vi "CalVision.vi"(10 "SerialPortIn":T1) -> (3 "SerialPortOut":T1)   [LabVIEW 2017, in "VisionHW.lvlib"]
uses:
  VisionHW.lvlib
  <vilib>/Rock Robotics/WPI/SerialPort/WPI_SerialPortRef.ctl
panel:
  out "Command":string
  in  "V Range":cluster{dbl, dbl}(slide) scale=0.0..255.0
  in  "S Range":cluster{dbl, dbl}(slide) scale=0.0..255.0
  in  "H Range":cluster{dbl, dbl}(slide) scale=0.0..255.0
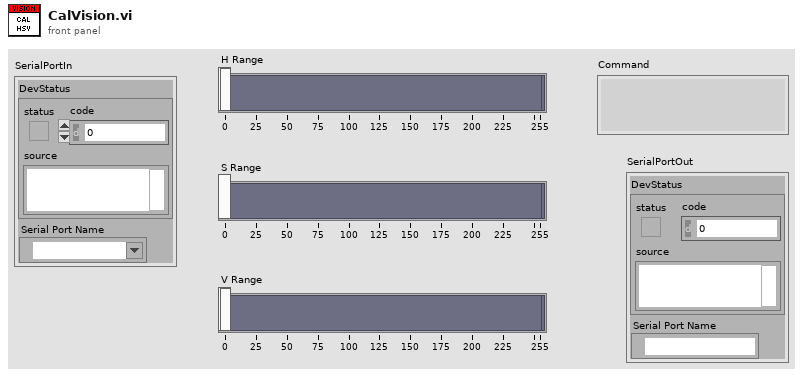
[diagram p1: front panel]
types:
  T1 = typedef "WPI_SerialPortRef.ctl" = cluster{"DevStatus":errorcluster, "Serial Port Name":refnum<visa-resource-name>}
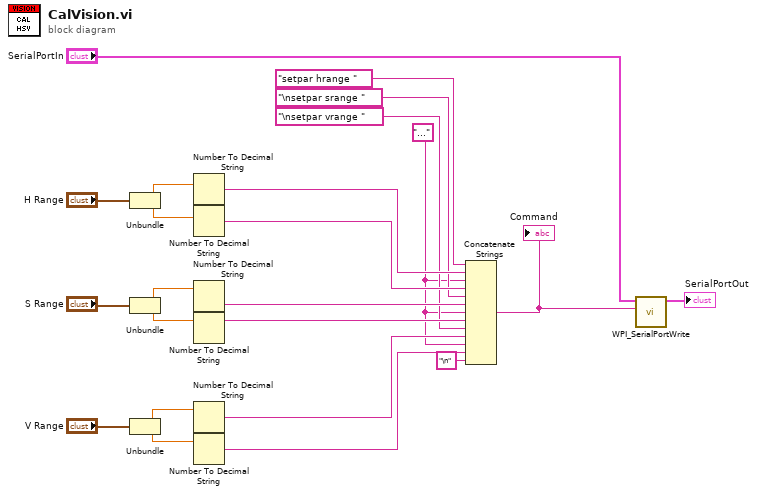
[diagram p0: block diagram]
diagram:
  w6 = "..." ("string")
  n1 = Unbundle("H Range") -> (w22:dbl, w19:dbl)
  n2 = Unbundle("S Range") -> (w15:dbl, w14:dbl)
  n3 = Unbundle("V Range") -> (w13:dbl, w12:dbl)
  n4 = Number To Decimal String(number=w22) -> (decimal integer string=w20:string)  [unwired: 1 in]
  n5 = Number To Decimal String(number=w19) -> (decimal integer string=w18:string)  [unwired: 1 in]
  n6 = Number To Decimal String(number=w15) -> (decimal integer string=w10:string)  [unwired: 1 in]
  n7 = Number To Decimal String(number=w14) -> (decimal integer string=w9:string)  [unwired: 1 in]
  n8 = Number To Decimal String(number=w13) -> (decimal integer string=w7:string)  [unwired: 1 in]
  n9 = Number To Decimal String(number=w12) -> (decimal integer string=w5:string)  [unwired: 1 in]
  n10 = Concatenate Strings("setpar hrange " ("string"), w20, w6, w18, "\nsetpar srange " ("string"), w10, w6, w9, "\nsetpar vrange " ("string"), w7, w6, w5, "\n" ("string")) -> (w3:string)
  "Command" <- w3
  n11 = call <vilib>:"WPI_SerialPortWrite.vi"("Buffer"=w3, "SerialPortRef"="SerialPortIn") -> ("SerialPortRef"=→"SerialPortOut":T1)  [unwired: 7 in, 2 out]
